vi "Init_Velocities-1.vi"() -> (0 "[OUT] Cluster with Velocities":T1)   [LabVIEW 2013]
panel:
  in  "Time Measurments \n(Unmoving)":i16[](array[numeric])
  in  "Time Measurments \n(Moving)":i32[](array[numeric])
  in  "Path Vel 2nd":dbl[](array[numeric])
  in  "Instant Vel 2nd":dbl[](array[numeric])
  in  "Path Vel 1st":dbl[](array[numeric])
  in  "Instant Vel 1st":dbl[](array[numeric])
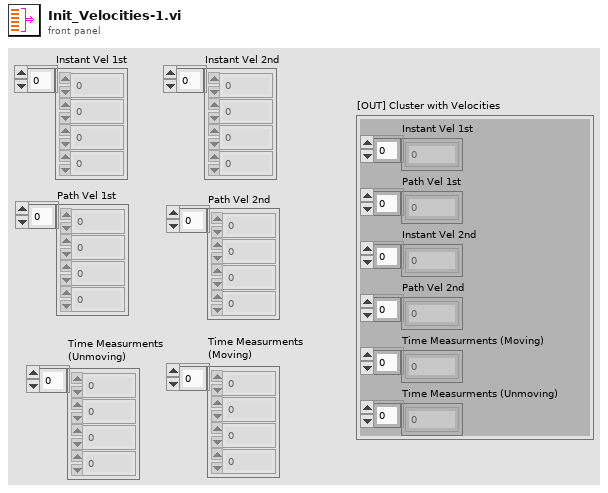
[diagram p1: front panel]
types:
  T1 = cluster{"Instant Vel 1st":dbl[], "Path Vel 1st ":dbl[], "Instant Vel 2nd  ":dbl[], "Path Vel 2nd":dbl[], "Time Measurments (Moving)":i32[], "Time Measurments (Unmoving) ":i16[]}
  T2 = cluster{"Instant Vel 1st":dbl[], "Path Vel 1st ":dbl[], "Instant Vel 2nd  ":dbl[], "Path Vel 2nd":dbl[], "Time Measurments \n(Moving)":i32[], "Time Measurments \n(Unmoving) ":i16[]}
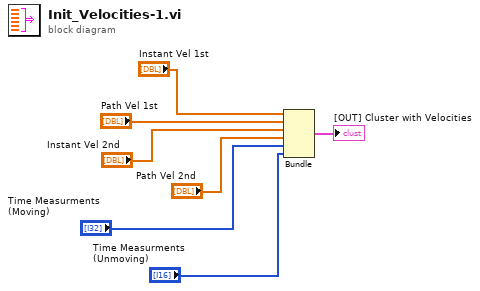
[diagram p0: block diagram]
diagram:
  n1 = Bundle("Instant Vel 1st"="Instant Vel 1st", "Path Vel 1st"="Path Vel 1st", "Instant Vel 2nd"="Instant Vel 2nd", "Path Vel 2nd"="Path Vel 2nd", "Time Measurments \n(Moving)"="Time Measurments \n(Moving)", "Time Measurments \n(Unmoving)"="Time Measurments \n(Unmoving)") -> (→"[OUT] Cluster with Velocities":T2)  [unwired: 1 in]
